vi "Save Panel Image to File.vi"(0 "vi path":path, 1 "visible area only":bool, 2 "Graphics file path":path, 3 "Image Depth":u16(ring)=2 items=["1-bit", "4-bit", "8-bit", "24-bit"], 4 "Graphic File Type":u16(ring) items=["BMP", "PNG", "JPEG"]) -> (5 "error out":errorcluster)   [LabVIEW 2019]
doc: "This VI demonstrates how to use the Get Panel Image method to save a VI's front panel in a JPEG, PNG, or BMP file.\n\nNOTE: This VI requires the shared libraries lvjpeg and lvpng, located in the LabVIEW\\Resource directory."
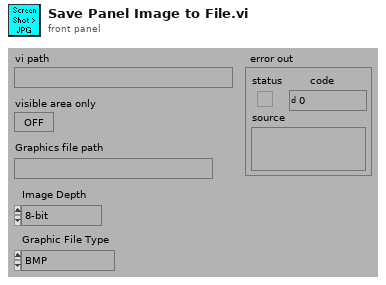
[diagram p1: front panel]
types:
  T1 = typedef "LVRectTypeDef.ctl" = cluster{"left":i16, "top":i16, "right":i16, "bottom":i16}
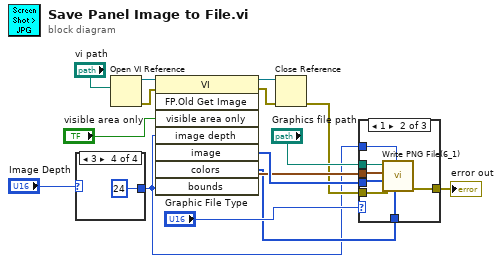
[diagram p0: block diagram]
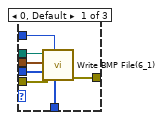
[diagram p2: hidden frame]
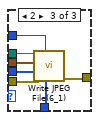
[diagram p3: hidden frame]
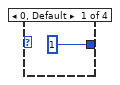
[diagram p4: hidden frame]
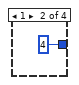
[diagram p5: hidden frame]
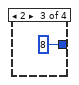
[diagram p6: hidden frame]
diagram:
  n1 = case shown="3" "Image Depth" {
    tunnel: [1 ("image depth") 4 ("image depth") 8 ("image depth") 24 ("image depth")] -> w1
    frame 0, Default {
    }
    frame 1 {
    }
    frame 2 {
    }
    frame 3 {
    }
  }
  n2 = Open VI Reference(vi path="vi path") -> (vi reference=w13:refnum<vi>, error out=w12:errorcluster)  [unwired: 5 in]
  n3 = invoke class="VI" method="FP.Old Get Image"(reference=w13, error in=w12, "visible area only"="visible area only", "image depth"=w1) -> (reference out=w15:refnum<vi>, error out=w14:errorcluster, "image"=w7:u8[], "colors"=w2:u32[], "bounds"=w5:T1)  [unwired: 4 in, 3 out]
  n4 = Close Reference(reference=w15, error in (no error)=w14) -> (error out=w4:errorcluster)
  n5 = case shown="1" "Graphic File Type" {
    tunnel: w7 -> [w26 w31 w39]
    tunnel: "Graphics file path" -> [w25 w33 w37]
    tunnel: w5 -> [w24 w32 w38]
    tunnel: w4 -> [w23 w30 w40]
    tunnel: [w22 w29 w36] -> w3
    tunnel: w2 -> [w20 w28 w34]
    tunnel: w1 -> [w21 w27 w35]
    frame 0, Default {
      n6 = call <vilib>:"Write BMP File(6_1).vi"("color table"=w20, "depth"=w21, "error in (no error)"=w23, "flattened image data"=w26, "rect"=w24, "path to BMP file"=w25) -> ("error out"=w22:errorcluster)  [unwired: 4 in, 1 out]
    }
    frame 1 {
      n7 = call <vilib>:"Write PNG File(6_1).vi"("color table"=w28, "depth"=w27, "error in (no error)"=w30, "flattened image data"=w31, "rect"=w32, "path to PNG file"=w33) -> ("error out"=w29:errorcluster)  [unwired: 4 in, 1 out]
    }
    frame 2 {
      n8 = call <vilib>:"Write JPEG File(6_1).vi"("color table"=w34, "depth"=w35, "error in (no error)"=w40, "flattened image data"=w39, "rect"=w38, "path to JPEG file"=w37) -> ("error out"=w36:errorcluster)  [unwired: 4 in, 1 out]
    }
  }
  "error out" <- w3
